vi "ViPER.vi"() -> ()   [LabVIEW 2022 SP3]
uses:
  <vilib>/picture/picture.llb/imagedata.ctl
  <userlib>/_OpenG.lib/file/file.llb/File Exists - Scalar__ogtk.vi
  Components/ViPER.lvlibp/ViPER.lvclass
panel:
  out "Label":string
  out "Picture":picture
  # ".net"
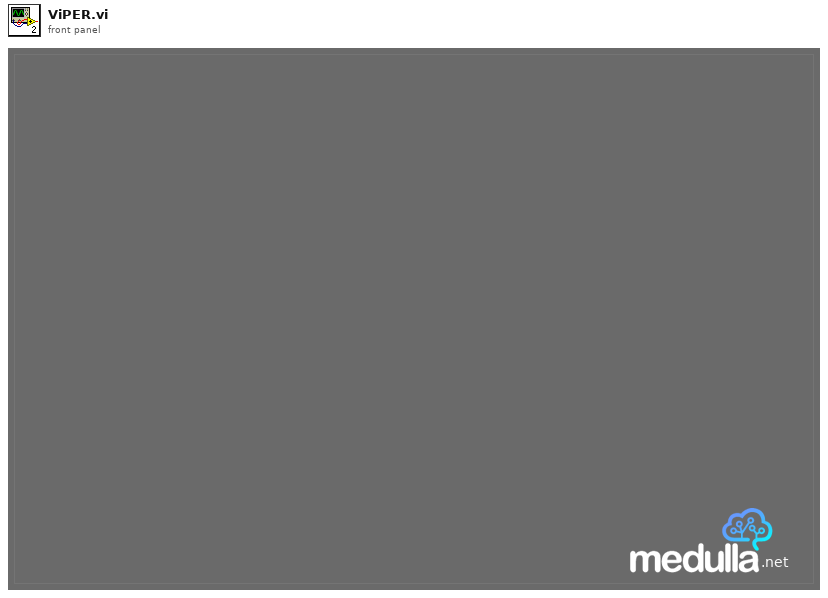
[diagram p1: front panel]
types:
  T1 = enum32{"Invalid", "Standard", "Closed", "Hidden", "Minimized", "Maximized"}
  T2 = typedef "imagedata.ctl" = cluster{"image type":i32, "image depth":i32, "image":u8[], "mask":u8[], "colors":u32[], "Rectangle":cluster{"left":i16, "top":i16, "right":i16, "bottom":i16}}
  T3 = enum32{"invalid app kind", "Development System", "Run Time System", "Student Edition", "Embedded LabVIEW", "Evaluation", "Custom"}
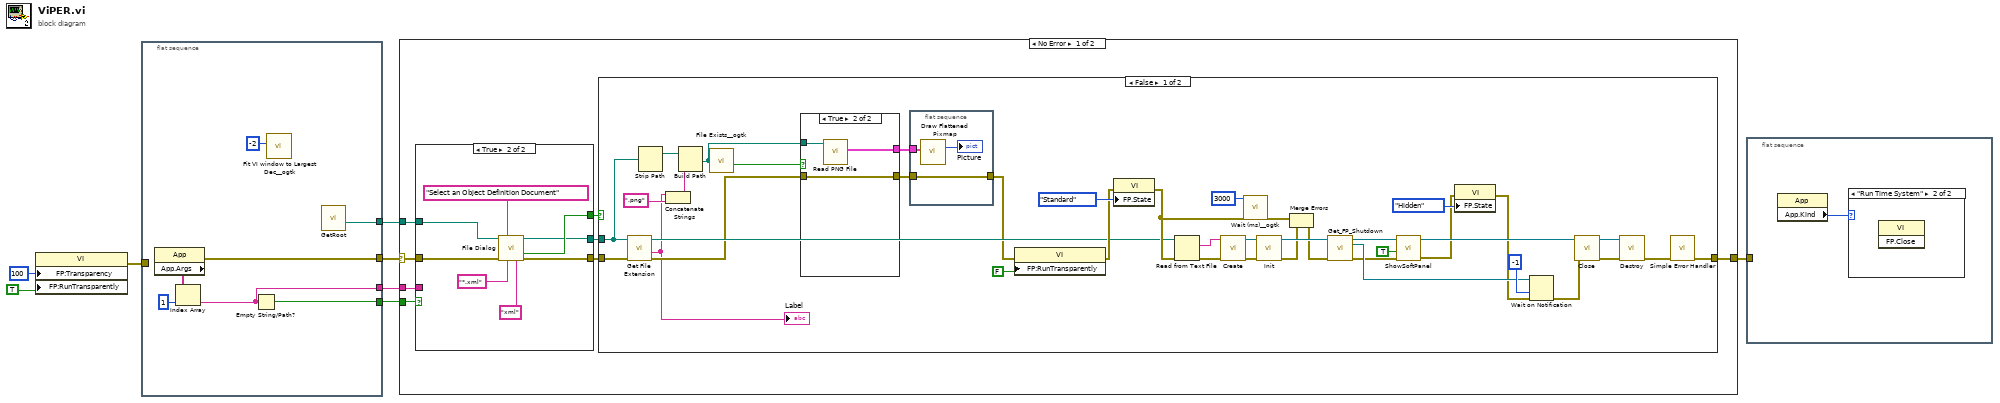
[diagram p0: block diagram]
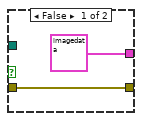
[diagram p2: hidden frame]
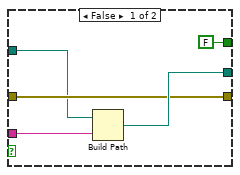
[diagram p4: hidden frame]
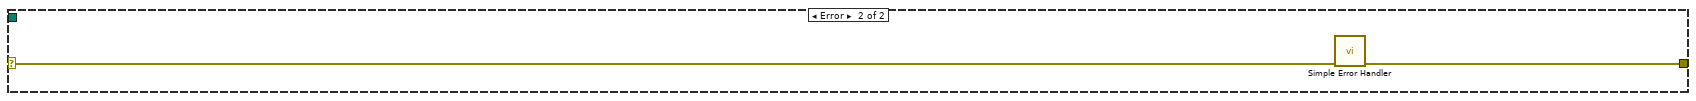
[diagram p5: hidden frame]
diagram:
  n1 = property class="VI"("FP:Transparency"=u8 100 ("Front Panel Window:Transparency"), "FP:RunTransparently"=TRUE ("Front Panel Window:Run VI Transparently")) -> (error out=w1:errorcluster)  [unwired: 2 in, 1 out]
  n2 = flat-sequence {
    tunnel: [w13] -> w8
    tunnel: [w11] -> w7
    tunnel: [w12] -> w6
    tunnel: [w10] -> w4
    tunnel: w1 -> [_]
    frame #0 {
      n3 = property class="App"() -> (error out=w10:errorcluster, "App.Args"=w15:string[])  [unwired: 2 in, 1 out]
      n4 = Index Array(array=w15, index=1) -> (element=w12:string)
      n5 = Empty String/Path?(string/path=w12) -> (empty?=w13:bool)
      n6 = call <userlib>:"Fit VI window to Largest Dec__ogtk.vi"("border spacing (2 px)"=-2) -> ()  [unwired: 5 in, 2 out]
      n7 = call "GetRoot.vi"() -> ("Root"=w11:path)  [unwired: 10 in, 1 out]
    }
  }
  n8 = case shown="No Error" w4 {
    selector: w4 -> [w16 w87]
    tunnel: w8 -> [w23 _]
    tunnel: w7 -> [w22 _]
    tunnel: w6 -> [w21 _]
    tunnel: [w20 w86] -> w5
    frame No Error {
      n9 = case shown="True" w23 {
        tunnel: w22 -> [w73 w78]
        tunnel: w21 -> [w77 _]
        tunnel: [w76 w80] -> w18
        tunnel: w16 -> [w74 w85]
        tunnel: [w74 w84] -> w19
        tunnel: [FALSE ("cancelled") w81] -> w17
        frame False {
          n10 = Build Path(base path=w73, name or relative path=w77) -> (appended path=w76:path)
        }
        frame True {
          n11 = call "File Dialog"("start path"=w78, "prompt"="Select an Object Definition Document", "error in"=w85, "pattern (all files)"="*.xml", "pattern label"="xml") -> ("selected path"=w80:path, "cancelled"=w81:bool, "error out"=w84:errorcluster)  [unwired: 7 in, 1 out]
        }
      }
      n12 = case shown="False" w17 {
        tunnel: [w41 w72] -> w20
        tunnel: w19 -> [w36 w72]
        tunnel: w18 -> [w34 _]
        frame False {
          n13 = call <vilib>:"Get File Extension.vi"("error in (no error)"=w36, "file"=w34) -> ("error out"=w30:errorcluster, "filename without extension"=w25:string, "dup file"=w35:path)  [unwired: 5 in, 2 out]
          "Label" <- w25
          n14 = Strip Path(path=w34) -> (stripped path=w33:path)  [unwired: 1 out]
          n15 = Concatenate Strings(w25, ".png" ("format string")) -> (w24:string)
          n16 = Build Path(base path=w33, name or relative path=w24) -> (appended path=w31:path)
          n17 = call-poly <userlib>:"File Exists__ogtk.vi"("file path"=w31) -> ("exists"=w32:bool)  [unwired: 6 in, 1 out]
          n18 = case shown="True" w32 {
            tunnel: w31 -> [_ w70]
            tunnel: w30 -> [w68 w71]
            tunnel: [w68 w71] -> w28
            tunnel: [T2 {"image type"=0, "image depth"=24, "image"=array[1279200 elements], "mask"=[], "colors"=[], "Rectangle"={"left"=0, "top"=0, "right"=800, "bottom"=533}} ("image data") w69] -> w29
            frame False {
            }
            frame True {
              n19 = call <vilib>:"Read PNG File.vi"("path to PNG file"=w70) -> ("image data"=w69:T2)  [unwired: 8 in, 2 out]
            }
          }
          n20 = flat-sequence {
            tunnel: w29 -> [w66]
            tunnel: w28 -> [w65]
            tunnel: [w65] -> w27
            frame #0 {
              n21 = call <vilib>:"Draw Flattened Pixmap.vi"("image data"=w66) -> ("new picture"=→"Picture":picture)  [unwired: 8 in]
            }
          }
          n22 = property class="VI"(error in=w27, "FP:RunTransparently"=FALSE ("Front Panel Window:Run VI Transparently")) -> (error out=w38:errorcluster)  [unwired: 1 in, 1 out]
          n23 = property class="VI"(error in=w38, "FP.State"=T1."Standard" ("Front Panel Window:State")) -> (error out=w37:errorcluster)  [unwired: 1 in, 1 out]
          n24 = Read from Text File(file (use dialog)=w35, error in=w37) -> (text=w50:string, error out=w51:errorcluster)  [unwired: 2 in, 2 out]
          n25 = call "Create.vi"("error in (no error)"=w51, "Config XML"=w50) -> ("error out"=w60:errorcluster, "reference out"=w61:refnum<class "ViPER.lvclass">)  [unwired: 8 in]
          n26 = call <userlib>:"Wait (ms)__ogtk.vi"("error in (no error)"=w37, "milliseconds to wait"=u32 3000) -> ("error out"=w44:errorcluster)  [unwired: 8 in, 1 out]
          n27 = call-dynamic "Init.vi"("error in (no error)"=w60, "reference in"=w61) -> ("error out"=w45:errorcluster, "reference out"=w59:refnum<class "ViPER.lvclass">)  [unwired: 8 in]
          n28 = Merge Errors(w44, w45) -> (w43:errorcluster)
          n29 = call "Get_FP_Shutdown.vi"("ViPER_Base in"=w59, "error in (no error)"=w43) -> ("ViPER_Base out"=w57:refnum<class "ViPER.lvclass">, "SoftFP_Shutdown"=w58:refnum<notifier>, "error out"=w56:errorcluster)  [unwired: 10 in, 1 out]
          n30 = call-dynamic "ShowSoftPanel.vi"("error in (no error)"=w56, "Floating"=TRUE, "Driver in"=w57) -> ("error out"=w47:errorcluster, "Driver out"=w55:refnum<class "ViPER.lvclass">)  [unwired: 6 in, 1 out]
          n31 = property class="VI"(error in=w47, "FP.State"=T1."Hidden" ("Front Panel Window:State")) -> (error out=w48:errorcluster)  [unwired: 1 in, 1 out]
          n32 = Wait on Notification(notifier=w58, timeout in ms (-1)=-1, error in (no error)=w48) -> (error out=w63:errorcluster)  [unwired: 1 in, 3 out]
          n33 = call-dynamic "Close.vi"("error in (no error)"=w63, "reference in"=w55) -> ("error out"=w54:errorcluster, "reference out"=w53:refnum<class "ViPER.lvclass">)  [unwired: 8 in]
          n34 = call "Destroy.vi"("error in (no error)"=w54, "reference in"=w53) -> ("error out"=w42:errorcluster)  [unwired: 9 in]
          n35 = call <vilib>:"Simple Error Handler.vi"("error in (no error)"=w42) -> ("error out"=w41:errorcluster)  [unwired: 4 in, 4 out]
        }
        frame True {
        }
      }
    }
    frame Error {
      n36 = call <vilib>:"Simple Error Handler.vi"("error in (no error)"=w87) -> ("error out"=w86:errorcluster)  [unwired: 4 in, 4 out]
    }
  }
  n37 = flat-sequence {
    tunnel: w5 -> [_]
    frame #0 {
      n38 = property class="App"() -> ("App.Kind"=w88:T3)  [unwired: 2 in, 2 out]
      n39 = case shown="\"Run Time System\"" w88 {
        frame "invalid app kind", Default {
        }
        frame "Run Time System" {
          n40 = invoke class="VI" method="FP.Close"() -> ()  [unwired: 3 in, 3 out]
        }
      }
    }
  }
